vi "Setup UI.vi"(8 "error in (no error)":errorcluster, 10 "Set UI to input? (F)":bool, 11 "Wavelength in":refnum<class "Wavelength Triax 550.lvclass">) -> (0 "error out":errorcluster, 3 "Wavelength out":refnum<class "Wavelength Triax 550.lvclass">)   [LabVIEW 2017, in "Wavelength Triax 550.lvclass"]
uses:
  Wavelength Triax 550.lvclass
  Instruments/Spectrometer Triax 550/JY-SPEX-TRIAX/controls.llb/Turret Position (TRIAX).ctl
  Wavelength Triax 550.lvclass/Wavelength Triax 550.ctl
  Instruments/Spectrometer Triax 550/Spectrometer Triax 550.lvclass
  C:/LabVIEW-programs/Instruments/Utility Classes/Scannable/Scannable.lvclass
  Instruments/Utility Classes/Scannable/Scannable.lvclass
  Instruments/Spectrometer Triax 550/JY-SPEX-TRIAX/JY-SPEX-TRIAX.lvlib
panel:
  in  "Shutter Toggle":bool
  in  "Current Grating":T2
  out "Current Wavelength":dbl[unit]
  in  "Set mirror (lateral)":bool
  in  "Go to first point":bool
  in  "Optimize":enum32{"Slits", "Step Size"}(radio)=enum."Step Size"
  out "Step size":dbl[unit] caption="Recommended step size\n(must enter above too)"
  in  "Lateral Exit":dbl[unit]
  in  "Axial Entrance":dbl[unit]
  # "Wavelength Scan Setup"
  # "NOTE: initial shutter value may be incorrect!  Toggle switch to set a definite value."
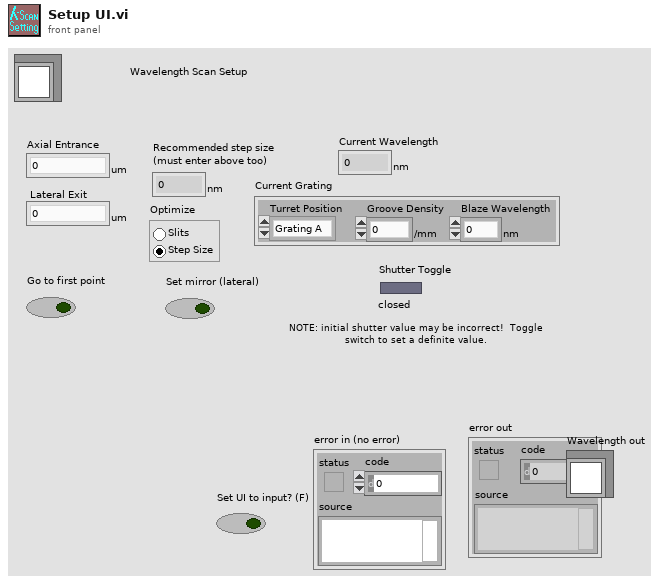
[diagram p1: front panel]
types:
  T1 = typedef "JY-SPEX-TRIAX.lvlib/Turret Position (TRIAX).ctl" = enum16{"Grating A", "Grating B", "Grating C"}
  T2 = cluster{"Turret Position":T1, "Groove Density":dbl[unit], "Blaze Wavelength":dbl[unit]}
  T3 = enum8{"Enabled", "Disabled", "Disabled and Grayed Out"}
  T4 = typedef "Scanner.lvclass/Range.ctl" = cluster{"xi":dbl, "xf":dbl, "dx":dbl, "Return to...?":bool, "Return to":dbl}
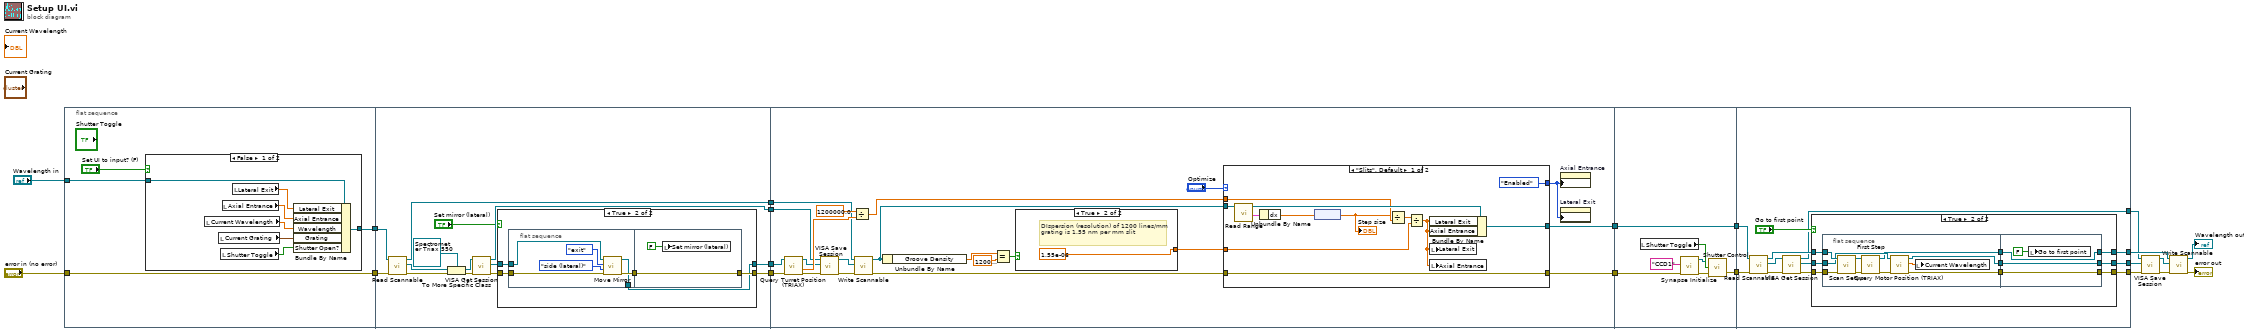
[diagram p0: block diagram]
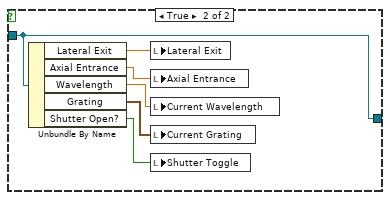
[diagram p2: hidden frame]
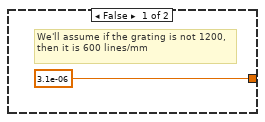
[diagram p4: hidden frame]
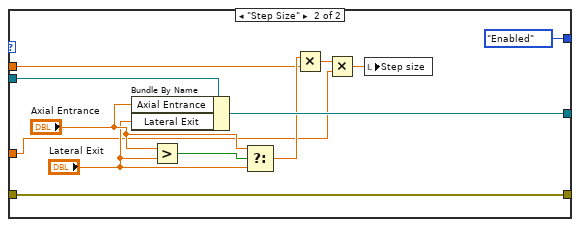
[diagram p5: hidden frame]
diagram:
  n1 = flat-sequence {
    tunnel: "Wavelength in" -> [w22]
    tunnel: "error in (no error)" -> [w24]
    tunnel: [w24] -> w12
    tunnel: [w21] -> w11
    tunnel: w12 -> [w45]
    tunnel: w11 -> [w46]
    tunnel: [w41] -> w10
    tunnel: [w42] -> w9
    tunnel: [w40] -> w8
    tunnel: [w38] -> w7
    tunnel: w10 -> [w74]
    tunnel: [w76] -> w6
    tunnel: [w75] -> w5
    tunnel: w9 -> [w73]
    tunnel: w8 -> [w72]
    tunnel: w7 -> [w71]
    tunnel: w6 -> [w115]
    tunnel: [w118] -> w4
    tunnel: w5 -> [w120]
    tunnel: [w120] -> w3
    tunnel: w4 -> [w124]
    tunnel: w3 -> [w128]
    tunnel: [w131] -> w17
    tunnel: [w130] -> w18
    tunnel: [w129] -> w14
    tunnel: [w121] -> w13
    frame #0 {
      n2 = case shown="False" "Set UI to input? (F)" {
        tunnel: w22 -> [w31 w32]
        tunnel: [w30 w32] -> w21
        frame False {
          n3 = local read "Current Wavelength"() -> (w27:dbl[unit])
          n4 = local read "Current Grating"() -> (w26:T2)
          n5 = local read "Shutter Toggle"() -> (w25:bool)
          n6 = local read "Axial Entrance"() -> (w28:dbl[unit])
          n7 = local read "Lateral Exit"() -> (w29:dbl[unit])
          n8 = Bundle By Name(cluster=w31, "Lateral Exit"=w29, "Axial Entrance"=w28, "Wavelength"=w27, "Grating"=w26, "Shutter Open?"=w25) -> (w30:refnum<class "Wavelength Triax 550.lvclass">)
        }
        frame True {
          n9 = Unbundle By Name(w32) -> ("Lateral Exit"=w37:dbl[unit], "Axial Entrance"=w36:dbl[unit], "Wavelength"=w35:dbl[unit], "Grating"=w34:T2, "Shutter Open?"=w33:bool)
          n10 = local write "Lateral Exit"(w37) -> ()
          n11 = local write "Axial Entrance"(w36) -> ()
          n12 = local write "Current Wavelength"(w35) -> ()
          n13 = local write "Current Grating"(w34) -> ()
          n14 = local write "Shutter Toggle"(w33) -> ()
        }
      }
    }
    frame #1 {
      n15 = call-dynamic "Read Scannable.vi"("error in (no error)"=w45, "Scanner.lvclass in"=w46) -> ("error out"=w51:errorcluster, "Scannable.lvclass"=w50:refnum<class "Scannable.lvclass">, "Scanner.lvclass out"=w38:refnum<class "Wavelength Triax 550.lvclass">)  [unwired: 7 out]
      n16 = To More Specific Class(target class=refnum<class "Spectrometer Triax 550.lvclass"> refnum ("Spectrometer Triax 550.lvclass"), reference=w50, error in=w51) -> (specific class reference=w47:refnum<class "Spectrometer Triax 550.lvclass">, error out=w48:errorcluster)
      n17 = call-dynamic "VISA Get Session.vi"("error in (no error)"=w48, "Instrument.lvclass in"=w47) -> ("error out"=w44:errorcluster, "VISA Resource Name"=w43:refnum<visa-resource-name>, "Instrument.lvclass out"=w42:refnum<class "Spectrometer Triax 550.lvclass">)  [unwired: 7 out]
      n18 = case shown="True" "Set mirror (lateral)" {
        tunnel: w44 -> [w53 w58]
        tunnel: [w53 w57] -> w41
        tunnel: w43 -> [w52 w55]
        tunnel: [w52 w54] -> w40
        frame False {
        }
        frame True {
          n19 = flat-sequence {
            tunnel: w58 -> [w62]
            tunnel: [w61] -> w56
            tunnel: w55 -> [w60]
            tunnel: [w59] -> w54
            tunnel: [w65] -> w57
            tunnel: w56 -> [w65]
            frame #0 {
              n20 = call "Move Mirror.vi"("error in (no error)"=w62, "position (side/lateral)"=enum16{"side (lateral)", "front (axial)"}."side (lateral)", "mirror (exit)"=enum16{"entrance", "exit"}."exit", "VISA resource name"=w60) -> ("error out"=w61:errorcluster, "VISA resource name out"=w59:refnum<visa-resource-name>)  [unwired: 1 in, 5 out]
            }
            frame #1 {
              n21 = local write "Set mirror (lateral)"(FALSE ("Set mirror (laterally)")) -> ()
            }
          }
        }
      }
    }
    frame #2 {
      n22 = call "Query Turret Position (TRIAX).vi"("error in (no error)"=w74, "VISA resource name"=w72) -> ("error out"=w82:errorcluster, "Groove Density"=w83:dbl[unit], "VISA resource name out"=w81:refnum<visa-resource-name>)  [unwired: 5 in, 2 out]
      n23 = call-dynamic "VISA Save Session.vi"("error in (no error)"=w82, "VISA Resource Name"=w81, "Instrument.lvclass in"=w73) -> ("error out"=w79:errorcluster, "Instrument.lvclass out"=w80:refnum<class "Spectrometer Triax 550.lvclass">)  [unwired: 7 out]
      n24 = Divide(x=dbl[unit] 1200000.0, y=w83) -> (x/y=w84:dbl)
      n25 = call-dynamic "Write Scannable.vi"("error in (no error)"=w79, "Scannable.lvclass"=w80, "Scanner.lvclass in"=w71) -> ("error out"=w85:errorcluster, "Scanner.lvclass out"=w86:refnum<class "Wavelength Triax 550.lvclass">)  [unwired: 7 out]
      n26 = Unbundle By Name(w86) -> ("Groove Density"=w70:dbl[unit])
      n27 = Equal?(x=w70, y=dbl[unit] 1200000.0) -> (x = y?=w68:bool)
      n28 = case shown="True" w68 {
        tunnel: [3.1e-06 1.55e-06] -> w67
        frame False {
          # "We'll assume if the grating is not 1200, then it is 600 lines/mm"
        }
        frame True {
          # "DIspersion (resolution) of 1200 lines/mm grating is 1.55 nm per mm slit"
        }
      }
      n29 = case shown="\"Slits\", Default" "Optimize" {
        tunnel: [w101 w112] -> w76
        tunnel: w85 -> [w101 w112]
        tunnel: w86 -> [w100 w103]
        tunnel: [w99 w111] -> w75
        tunnel: [T3."Enabled" ("Disabled") T3."Enabled" ("Disabled")] -> w78
        tunnel: w84 -> [w92 w104]
        tunnel: w67 -> [w90 w102]
        frame "Slits", Default {
          n30 = call-dynamic "Read Range.vi"("Scanner.lvclass in"=w100) -> ("Range"=w96:T4, "Scanner.lvclass out"=w97:refnum<class "Wavelength Triax 550.lvclass">)  [unwired: 5 in, 4 out]
          n31 = Unbundle By Name(w96) -> ("dx"=w95:dbl)
          n32 = node(w95) -> (w91:dbl[unit])
          "Step size" <- w91
          n33 = Divide(x=w91, y=w92) -> (x/y=w93:dbl[unit])
          n34 = Divide(x=w93, y=w90) -> (x/y=w98:dbl[unit])
          n35 = Bundle By Name(cluster=w97, "Lateral Exit"=w98, "Axial Entrance"=w98) -> (w99:refnum<class "Wavelength Triax 550.lvclass">)
          n36 = local write "Lateral Exit"(w98) -> ()
          n37 = local write "Axial Entrance"(w98) -> ()
        }
        frame "Step Size" {
          n38 = Bundle By Name(cluster=w103, "Axial Entrance"="Axial Entrance", "Lateral Exit"="Lateral Exit") -> (w111:refnum<class "Wavelength Triax 550.lvclass">)
          n39 = Greater?(x="Axial Entrance", y="Lateral Exit") -> (0:w113:bool)
          n40 = Select(t="Axial Entrance", s=w113, f="Lateral Exit") -> (s? t:f=w105:dbl[unit])
          n41 = Multiply(x=w105, y=w104) -> (x*y=w106:dbl[unit])
          n42 = Multiply(x=w106, y=w102) -> (x*y=w107:dbl[unit])
          n43 = local write "Step size"(w107) -> ()
        }
      }
      n44 = property on="Axial Entrance" class="DigNum (strict)"("DisabledEnum"=w78) -> ()  [unwired: 2 in, 2 out]
      n45 = property on="Lateral Exit" class="DigNum (strict)"("DisabledEnum"=w78) -> ()  [unwired: 2 in, 2 out]
    }
    frame #3 {
      n46 = local read "Shutter Toggle"() -> (w119:bool)
      n47 = call "Synapse Initialize.vi"("error in (no error)"=w115, "Unique id"="CCD1") -> ("error out"=w114:errorcluster, "JYCCDLib.IJYCCDReqd"=w116:refnum<k7>)  [unwired: 1 in, 7 out]
      n48 = call "Shutter Control.vi"("input error"=w114, "Shutter"=w119, "JYCCDLib.IJYCCDReqd"=w116) -> ("error out"=w118:errorcluster)  [unwired: 1 out]
    }
    frame #4 {
      n49 = call-dynamic "Read Scannable.vi"("error in (no error)"=w124, "Scanner.lvclass in"=w128) -> ("error out"=w123:errorcluster, "Scannable.lvclass"=w127:refnum<class "Scannable.lvclass">, "Scanner.lvclass out"=w126:refnum<class "Wavelength Triax 550.lvclass">)  [unwired: 7 out]
      n50 = call-dynamic "VISA Get Session.vi"("error in (no error)"=w123, "Instrument.lvclass in"=w127) -> ("error out"=w122:errorcluster, "VISA Resource Name"=w125:refnum<visa-resource-name>, "Instrument.lvclass out"=w121:refnum<class "Scannable.lvclass">)  [unwired: 7 out]
      n51 = case shown="True" "Go to first point" {
        tunnel: w126 -> [w134 w144]
        tunnel: w122 -> [w135 w143]
        tunnel: [w135 w142] -> w131
        tunnel: [w133 w140] -> w130
        tunnel: [w134 w137] -> w129
        tunnel: w125 -> [w133 w138]
        frame False {
        }
        frame True {
          n52 = flat-sequence {
            tunnel: w144 -> [w151]
            tunnel: w143 -> [w154]
            tunnel: [w150] -> w141
            tunnel: [w148] -> w139
            tunnel: w138 -> [w147]
            tunnel: [w145] -> w136
            tunnel: [w158] -> w142
            tunnel: w141 -> [w158]
            tunnel: [w156] -> w140
            tunnel: w139 -> [w156]
            tunnel: [w155] -> w137
            tunnel: w136 -> [w155]
            frame #0 {
              n53 = call-dynamic "Scan Setup.vi"("error in (no error)"=w154, "Wavelength in"=w151) -> ("error out"=w153:errorcluster, "Wavelength out"=w152:refnum<class "Wavelength Triax 550.lvclass">)  [unwired: 8 in]
              n54 = call-dynamic "First Step.vi"("error in (no error)"=w153, "Wavelength.lvclass in"=w152) -> ("error out"=w146:errorcluster, "Wavelength.lvclass out"=w145:refnum<class "Wavelength Triax 550.lvclass">)  [unwired: 7 in, 1 out]
              n55 = call "Query Motor Position (TRIAX).vi"("error in (no error)"=w146, "VISA resource name"=w147) -> ("error out"=w150:errorcluster, "wavelength"=w149:dbl[unit], "VISA resource name out"=w148:refnum<visa-resource-name>)  [unwired: 1 in, 6 out]
              n56 = local write "Current Wavelength"(w149) -> ()
            }
            frame #1 {
              n57 = local write "Go to first point"(FALSE ("Go to first point")) -> ()
            }
          }
        }
      }
    }
  }
  n58 = call-dynamic "VISA Save Session.vi"("error in (no error)"=w17, "VISA Resource Name"=w18, "Instrument.lvclass in"=w13) -> ("error out"=w16:errorcluster, "Instrument.lvclass out"=w1:refnum<class "Scannable.lvclass">)  [unwired: 7 out]
  n59 = call-dynamic "Write Scannable.vi"("error in (no error)"=w16, "Scannable.lvclass"=w1, "Scanner.lvclass in"=w14) -> ("error out"=→"error out":errorcluster, "Scanner.lvclass out"=→"Wavelength out":refnum<class "Wavelength Triax 550.lvclass">)  [unwired: 7 out]
